vi "Put_I64_PV-I.vi"(8 "Error in (no error)":errorcluster, 10 "Value":i64, 11 "CA Lab data":T2) -> (0 "Error out":errorcluster, 1 "PV error":errorcluster, 2 "Status":bool, 3 "PV Name (dup)":string)   [LabVIEW 2018]
doc: "This is a polymorphic VI for setting values of EPICS variables.\n\nINPUT:\n <b>PV name(s)</b>\n name of EPICS variable\n <b>value(s)</b>\n Boolean value OR Double value OR Double array OR String array\n <b>timeout</b>\n optional\n timeout for Channel Access requests\n <b>error in</b>\n <b>buffer size (since version 1.3 without function)</b>\n <b>synchronous</b>\n optional\n TRUE=synchronous; FALSE=asynchronous\n synchronous = writes value(s) after waiting for end of record processing\n <b>ValueSetsInColumns</b>\n optional\n TRUE = use columns for value sets instead of rows\n\nOUTPUT:\n <b>PV name(s)</b>\n name of EPICS variable\n </b>status</b>\n FALSE: request successful\n TRUE: warnings or errors\n <b>errors</b>\n resulting errors of all put commands\n <b>error out</b>\n global io error"
uses:
  <userlib>/caLab/PV Info.ctl
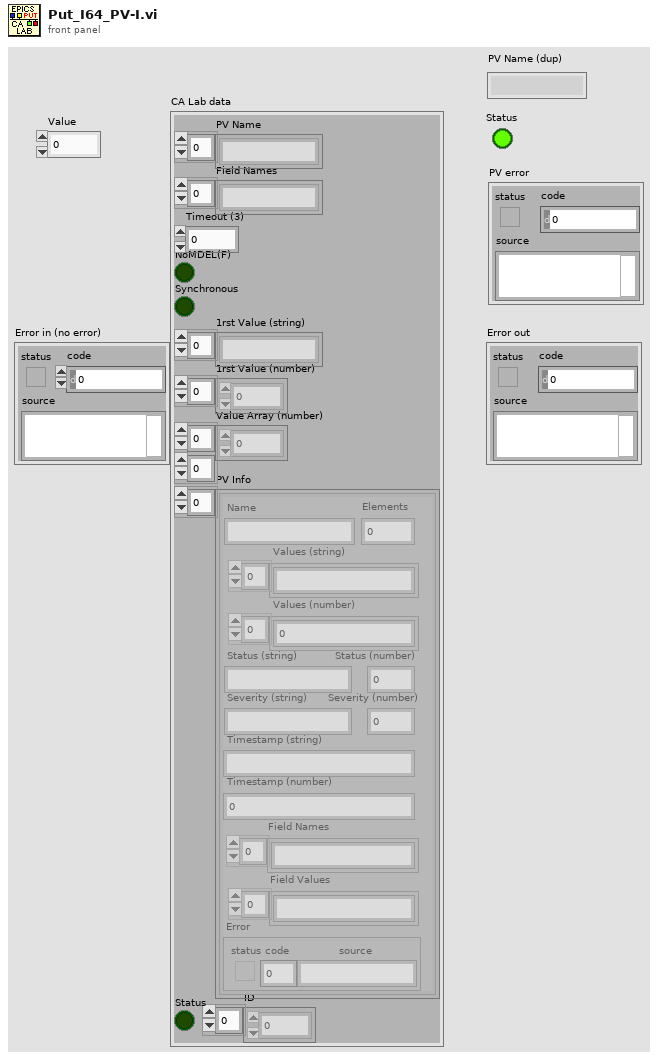
[diagram p1: front panel]
types:
  T1 = typedef "PV Info.ctl" = cluster{"Name":string, "Elements":i32, "Values (string)":string[], "Values (number)":dbl[], "Status (string)":string, "Status (number)":i16, "Severity (string)":string, "Severity (number)":i16, "Timestamp (string)":string, "Timestamp (number)":i32, "Field Names":string[], "Field Values":string[], "Error":errorcluster}
  T2 = cluster{"PV Name":string[], "Field Names":string[], "Timeout (3)":dbl, "NoMDEL(F)":bool, "Synchronous":bool, "1rst Value (string)":string[], "1rst Value (number)":dbl[], "Value Array (number)":dbl[][], "PV Info":T1[], "Status":bool, "ID":u64[]}
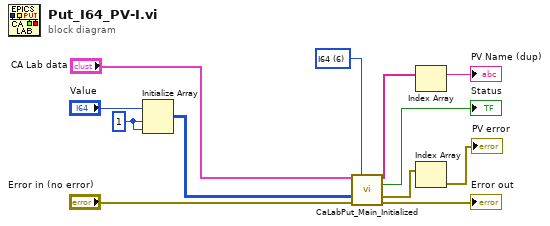
[diagram p0: block diagram]
diagram:
  w7 = 1 ("dimension size")
  w12 = 6 items=["String", "SGL", "DBL", "I8", "I16", "I32", "I64"] ("data type")
  n1 = Initialize Array("Value", w7, w7) -> (w6:i64[][])
  n2 = call <userlib>:"CaLabPut_Main_Initialized.vi"("CA Lab data"="CA Lab data", "Data Type"=w12, "Values [I64]"=w6, "Error in (no error)"="Error in (no error)") -> ("PV Names (dup)"=w2:string[], "Status"=→"Status":bool, "PV Errors"=w4:errorcluster[], "Error out"=→"Error out":errorcluster)  [unwired: 8 in]
  n3 = Index Array(array=w2) -> (element=→"PV Name (dup)":string)  [unwired: 1 in]
  n4 = Index Array(array=w4) -> (element=→"PV error":errorcluster)  [unwired: 1 in]
